vi "Save Module to Slot.vi"(8 "error in":errorcluster, 10 "RSI module in":refnum<class "RSI Module.lvclass">, 11 "slot ref in":T1 format="%.0x") -> (0 "error out":errorcluster, 2 "RSI module out":refnum<class "RSI Module.lvclass">, 3 "slot ref out":T1 format="%.0x")   [LabVIEW 2019, in "Scan Engine Scripting.lvlib"]
uses:
  Scan Engine Scripting.lvlib
  SEECD System Explorer.lvlib
  Modules.lvlibp/RSI Module/RSI Module.lvclass
  Modules.lvlibp/1abvi3w/vi.lib/NI VeriStand/Custom Device API/Custom Device Item Ref.ctl
  Modules.lvlibp/1abvi3w/vi.lib/NI VeriStand/Custom Device API/Custom Device API.lvlib
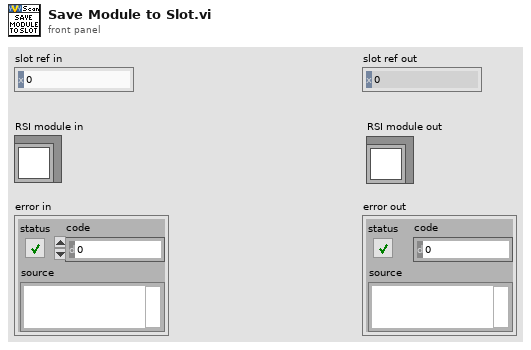
[diagram p1: front panel]
types:
  T1 = typedef "Modules.lvlibp/Custom Device API.lvlib/Custom Device Item Ref.ctl" = u64
  T2 = typedef "Custom Device API.lvlib/Custom Device Item Ref.ctl" = u64
  T3 = typedef "Modules.lvlibp/RSI Module.lvclass/Module Models.ctl" = enum16{"Empty", "NI 9201", "NI 9203", "NI 9205", "NI 9206", "NI 9207", "NI 9208", "NI 9209", "NI 9210", "NI 9211", "NI 9212", "NI 9213", "NI 9214", "NI 9215", "NI 9216", "NI 9217", "NI 9219", "NI 9220", "NI 9221", "NI 9222", "NI 9223", "NI 9224", "NI 9225", "NI 9226", "NI 9227", "NI 9228", "NI 9229", "NI 9233", "NI 9234", "NI 9235", "NI 9236", "NI 9237", "NI 9239", "NI 9242", "NI 9244", "NI 9253", "NI 9263", "NI 9264", "NI 9265", "NI 9266", "NI 9269", "NI 9344", "NI 9350", "NI 9375", "NI 9401", "NI 9402", "NI 9403", "NI 9411", "NI 9421", "NI 9422", "NI 9423", "NI 9425", "NI 9426", "NI 9435", "NI 9436", "NI 9437", "NI 9472", "NI 9474", "NI 9475", "NI 9476", "NI 9477", "NI 9478", "NI 9481", "NI 9482", "NI 9485"}
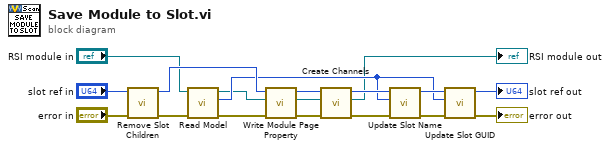
[diagram p0: block diagram]
diagram:
  n1 = call "Remove Slot Children.vi"("error in"="error in", "slot ref in"="slot ref in") -> ("error out"=w16:errorcluster, "slot ref out"=w18:T2)  [unwired: 8 in]
  n2 = call "Read Model.vi"("error in (no error)"=w16, "RSI Module in"="RSI module in") -> ("error out"=w8:errorcluster, "Model"=w11:T3, "RSI Module out"=w7:refnum<class "RSI Module.lvclass">)  [unwired: 7 in]
  n3 = call "Write Module Page Property.vi"("error in (no error)"=w8, "RSI Module"=w7, "Node Ptr In"=w18) -> ("error out"=w5:errorcluster, "RSI Module out"=w3:refnum<class "RSI Module.lvclass">, "Node Ptr Out"=w10:T1)  [unwired: 6 in]
  n4 = call-dynamic "Create Channels.vi"("error in (no error)"=w5, "RSI Module in"=w3, "Parent Ref in"=w10) -> ("error out"=w4:errorcluster, "RSI Module out"=→"RSI module out":refnum<class "RSI Module.lvclass">, "Parent Ref out"=w12:T1)  [unwired: 6 in]
  n5 = call "Update Slot Name.vi"("error in"=w4, "module"=w11, "slot ref in"=w12) -> ("error out"=w6:errorcluster, "slot ref out"=w13:T2)  [unwired: 6 in, 1 out]
  n6 = call "Update Slot GUID.vi"("error in"=w6, "module model"=w11, "slot ref in"=w13) -> ("error out"=→"error out":errorcluster, "slot ref out"=→"slot ref out":T2)  [unwired: 7 in]
